vi "Configure Trace Point.vi"(0 "VISA resource name":refnum<visa-resource-name>, 5 "Trace Points (12:10001)":i32(ring)=12 items=["11", "21", "41", "51", "101", "201", "251", "401", "501", "1001", "2001", "5001", "10001"], 11 "error in (no error)":errorcluster) -> (4 "VISA resource name out":refnum<visa-resource-name>, 15 "error out":errorcluster)   [LabVIEW 2023, in "Anritsu Signal Analyzer Series.lvlib"]
doc: "Configures the number of trace display points of the spectrum analyzer."
uses:
  Anritsu Signal Analyzer Series.lvlib
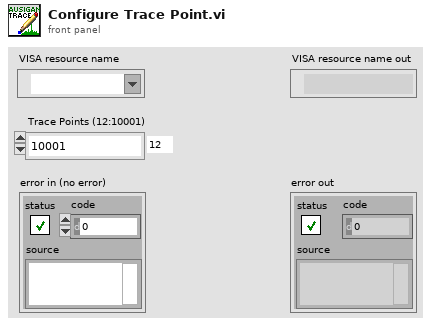
[diagram p1: front panel]
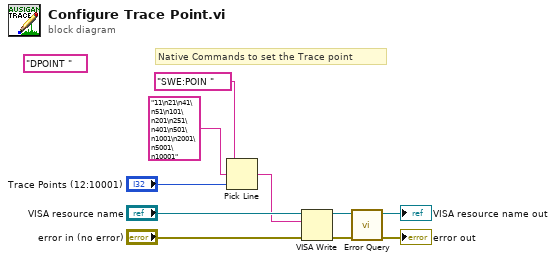
[diagram p0: block diagram]
diagram:
  (unwired) "DPOINT "
  # "Native Commands to set the Trace point"
  n1 = Pick Line(string ("")="SWE:POIN ", multi-line string="11\n21\n41\n51\n101\n201\n251\n401\n501\n1001\n2001\n5001\n10001" ("複数行文字列"), line index="Trace Points (12:10001)") -> (output string=w1:string)
  n2 = VISA Write(VISA resource name="VISA resource name", write buffer=w1, error in (no error)="error in (no error)") -> (VISA resource name out=w4:refnum<visa-resource-name>, error out=w5:errorcluster)  [unwired: 1 out]
  n3 = call "Error Query.vi"("error in (no error)"=w5, "VISA resource name"=w4) -> ("error out"=→"error out":errorcluster, "VISA resource name out"=→"VISA resource name out":refnum<visa-resource-name>)  [unwired: 6 in, 2 out]
